vi "Jeffress_model_v008-DESKTOP-66GCGQA.vi"() -> ()   [LabVIEW 2019]
panel:
  out "Elapsed time 2":dbl caption="Get Start Time (s)"
  out "new picture":picture
  out "Left - Right":dbl
  out "Elapsed time 1":dbl caption="Get Start Time (s)"
  in  "stop":bool
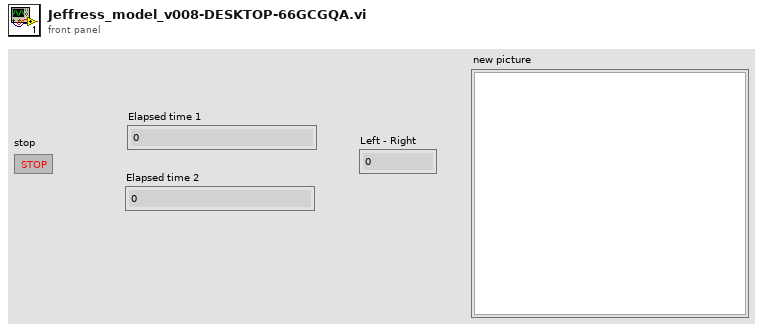
[diagram p1: front panel]
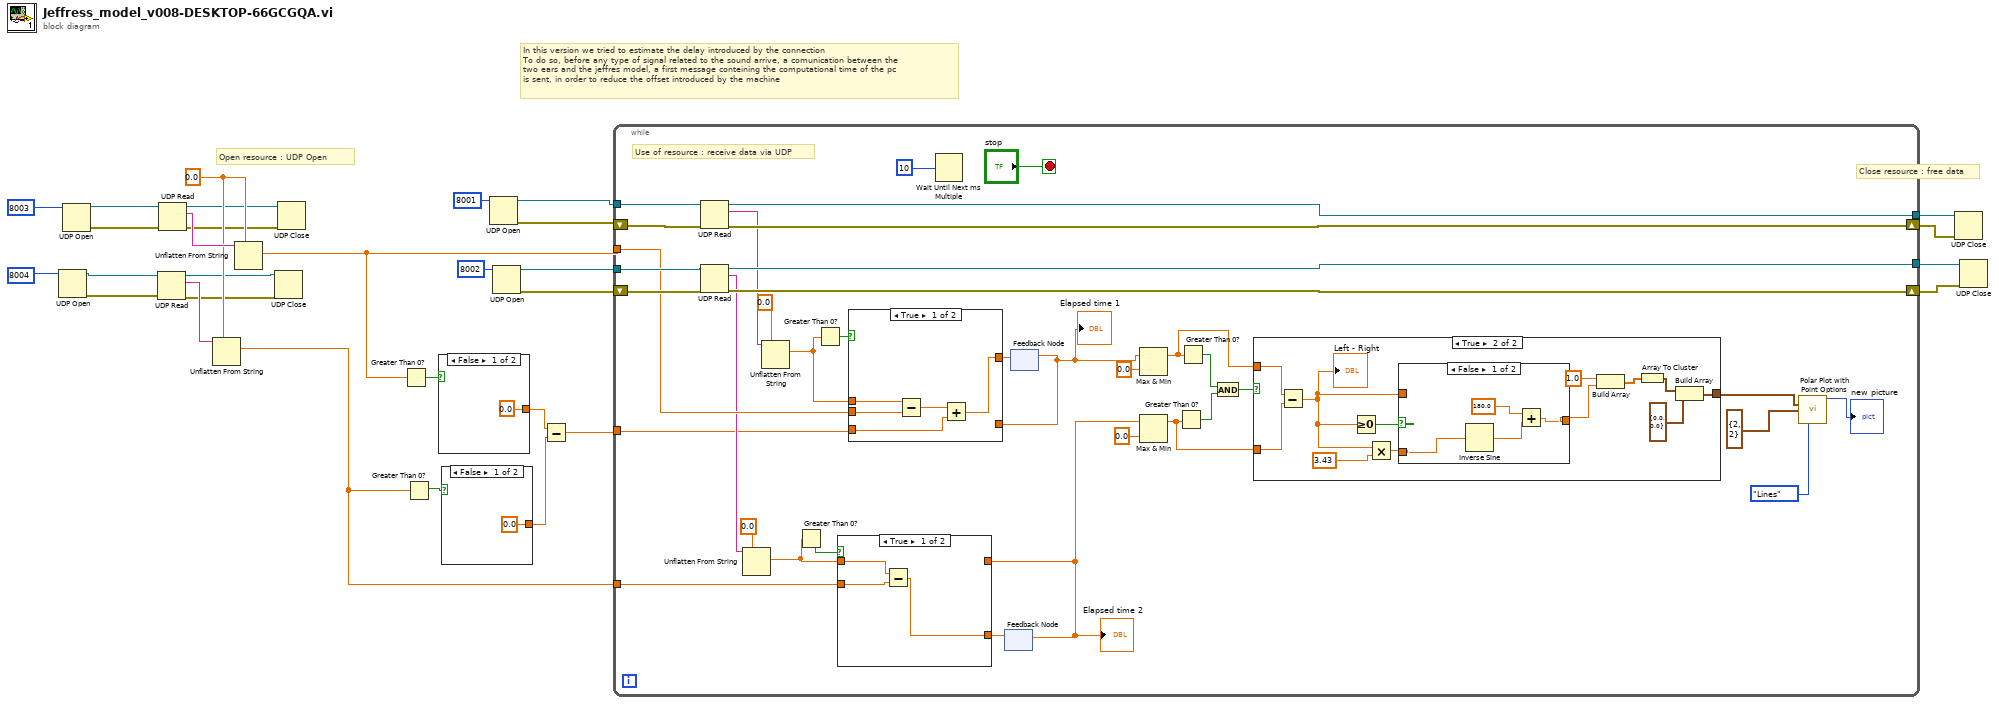
[diagram p0: block diagram]
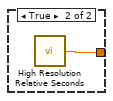
[diagram p2: hidden frame]
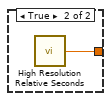
[diagram p3: hidden frame]
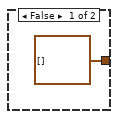
[diagram p5: hidden frame]
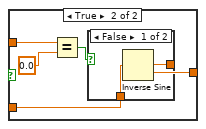
[diagram p6: hidden frame]
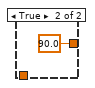
[diagram p7: hidden frame]
diagram:
  w18 = 0.0
  # "In this version we tried to estimate the delay introduced by the connection\nTo do so, before any type of signal related to the sound arrive, a comunication between the\ntwo ears and the jeffres model, a first message conteining the computational time of the pc\nis sent, in order to reduce the offset introduced by the machine"
  # "Close resource : free data"
  # "Open resource : UDP Open"
  n1 = UDP Open(11:u16 8004) -> (port=w22:refnum<k16>, 0:w21:errorcluster)  [unwired: 4 in, 1 out]
  n2 = UDP Open(11:u16 8003) -> (port=w24:refnum<k16>, 0:w23:errorcluster)  [unwired: 4 in, 1 out]
  n3 = UDP Read(connection ID=w22, 8:w21) -> (data out=w19:string, error out=w14:errorcluster, 3:w15:refnum<k16>)  [unwired: 2 in, 2 out]
  n4 = UDP Read(connection ID=w24, 8:w23) -> (data out=w20:string, error out=w16:errorcluster, 3:w17:refnum<k16>)  [unwired: 2 in, 2 out]
  n5 = Unflatten From String(type=w18, binary string=w19) -> (value=w4:dbl)  [unwired: 3 in, 2 out]
  n6 = Unflatten From String(type=w18, binary string=w20) -> (value=w6:dbl)  [unwired: 3 in, 2 out]
  n7 = UDP Close(connection ID=w15, 8:w14) -> ()  [unwired: 2 out]
  n8 = UDP Close(connection ID=w17, 8:w16) -> ()  [unwired: 2 out]
  n9 = Greater Than 0?(x=w6) -> (x > 0?=w7:bool)
  n10 = Greater Than 0?(x=w4) -> (x > 0?=w5:bool)
  n11 = case shown="False" w7 {
    tunnel: [0.0 ("relative seconds") w32] -> w3
    frame False {
    }
    frame True {
      n12 = call <vilib>:"High Resolution Relative Seconds.vi"() -> ("relative seconds"=w32:dbl)
    }
  }
  n13 = case shown="False" w5 {
    tunnel: [0.0 ("relative seconds") w34] -> w2
    frame False {
    }
    frame True {
      n14 = call <vilib>:"High Resolution Relative Seconds.vi"() -> ("relative seconds"=w34:dbl)
    }
  }
  n15 = UDP Open(11:u16 8001 ("port")) -> (port=w13:refnum<k16>, 0:w12:errorcluster)  [unwired: 4 in, 1 out]
  n16 = UDP Open(11:u16 8002 ("port")) -> (port=w11:refnum<k16>, 0:w10:errorcluster)  [unwired: 4 in, 1 out]
  n17 = Subtract(x=w3, y=w2) -> (x-y=w1:dbl)
  n18 = while {
    tunnel: w13 -> [w66]
    tunnel: [w65] -> w29
    shift-right: [w68] -> w30
    shift-left: w12 -> [w67]
    tunnel: w11 -> [w54]
    tunnel: [w52] -> w25
    shift-right: [w53] -> w26
    shift-left: w10 -> [w51]
    tunnel: w4 -> [w43]
    tunnel: w6 -> [w42]
    tunnel: w1 -> [w35]
    stop <- "stop" stop-if-true
    # "Use of resource : receive data via UDP"
    n19 = UDP Read(connection ID=w66, 8:w67) -> (data out=w46:string, error out=w68:errorcluster, 3:w65:refnum<k16>)  [unwired: 2 in, 2 out]
    n20 = UDP Read(connection ID=w54, 8:w51) -> (data out=w37:string, error out=w53:errorcluster, 3:w52:refnum<k16>)  [unwired: 2 in, 2 out]
    n21 = Unflatten From String(type=0.0, binary string=w37) -> (value=w44:dbl)  [unwired: 3 in, 2 out]
    n22 = Unflatten From String(type=0.0, binary string=w46) -> (value=w41:dbl)  [unwired: 3 in, 2 out]
    n23 = Greater Than 0?(x=w44) -> (x > 0?=w36:bool)
    n24 = Greater Than 0?(x=w41) -> (x > 0?=w45:bool)
    n25 = Wait Until Next ms Multiple(millisecond multiple=u32 10) -> ()  [unwired: 1 out]
    n26 = feedback #1() -> (w38:dbl)  [unwired: 1 in]
    "Elapsed time 2" <- w38
    n27 = case shown="True" w36 {
      tunnel: [w102 w105] -> w49
      tunnel: w38 -> [_ w105]
      tunnel: w44 -> [w104 _]
      tunnel: w43 -> [w103 _]
      frame True {
        n28 = Subtract(x=w104, y=w103) -> (x-y=w102:dbl)
      }
      frame False, Default {
      }
    }
    n29 = feedback-in #1(w49) -> ()
    n30 = feedback #2() -> (w47:dbl)  [unwired: 1 in]
    "Elapsed time 1" <- w47
    n31 = case shown="True" w45 {
      tunnel: [w72 w76] -> w48
      tunnel: w47 -> [_ w76]
      tunnel: w42 -> [w75 _]
      tunnel: w41 -> [w74 _]
      tunnel: w35 -> [w71 _]
      frame True {
        n32 = Subtract(x=w74, y=w75) -> (x-y=w73:dbl)
        n33 = Add(x=w73, y=w71) -> (x+y=w72:dbl)
      }
      frame False {
      }
    }
    n34 = feedback-in #2(w48) -> ()
    n35 = Max & Min(x=w47, y=0.0) -> (max(x,y)=w59:dbl)  [unwired: 1 out]
    n36 = Max & Min(x=w38, y=0.0) -> (max(x,y)=w60:dbl)  [unwired: 1 out]
    n37 = Greater Than 0?(x=w60) -> (x > 0?=w61:bool)
    n38 = Greater Than 0?(x=w59) -> (x > 0?=w62:bool)
    n39 = And(x=w62, y=w61) -> (x .and. y?=w50:bool)
    n40 = case shown="True" w50 {
      tunnel: w59 -> [_ w88]
      tunnel: w60 -> [_ w89]
      tunnel: [cluster{"[0]":dbl, "[1]":dbl}[] [] w83] -> w58
      frame False {
      }
      frame True {
        n41 = Subtract(x=w88, y=w89) -> (x-y=w78:dbl)
        "Left - Right" <- w78
        n42 = Greater Or Equal To 0?(x=w78) -> (x >= 0?=w87:bool)
        n43 = Multiply(x=w78, y=3.43) -> (x*y=w82:dbl)
        n44 = case shown="False" w87 {
          tunnel: w82 -> [w93 w97]
          tunnel: [w92 w98] -> w81
          tunnel: w78 -> [_ w94]
          frame False {
            n45 = Inverse Sine(1:w93) -> (0:w91:dbl)
            n46 = Add(x=180.0, y=w91) -> (x+y=w92:dbl)
          }
          frame True {
            n47 = Equal?(x=w94, y=0.0 ("x")) -> (x = y?=w96:bool)
            n48 = case shown="False" w96 {
              tunnel: [w100 90.0] -> w98
              tunnel: w97 -> [w99 _]
              frame False {
                n49 = Inverse Sine(1:w99) -> (0:w100:dbl)
              }
              frame True {
              }
            }
          }
        }
        n50 = Build Array(1.0 ("element"), w81) -> (w85:dbl[])
        n51 = Array To Cluster(array=w85) -> (cluster=w84:cluster{"[0]":dbl, "[1]":dbl})
        n52 = Build Array(w84, cluster{"[0]":dbl, "[1]":dbl} {"[0]"=0.0, "[1]"=0.0} ("element")) -> (w83:cluster{"[0]":dbl, "[1]":dbl}[])
      }
    }
    n53 = call <vilib>:"Polar Plot with Point Options.vi"("data array [mag, phase (deg)]"=w58, "top left point(0, 0)"=cluster{"x":i16, "y":i16} {"x"=2, "y"=2}, "Lines/Points"=enum16{"Lines", "Points"}."Lines") -> ("new picture"=→"new picture":picture)  [unwired: 12 in]
  }
  n54 = UDP Close(connection ID=w29, 8:w30) -> ()  [unwired: 2 out]
  n55 = UDP Close(connection ID=w25, 8:w26) -> ()  [unwired: 2 out]
